vi "Rotation_CreateAngleDegrees.vi"(11 "Angle_Degrees":dbl) -> (3 "ROTATION":T1 {"SIN" format="%13.4f"; "COS" format="%13.4f"; "VALUE" format="%13.4f"})   [LabVIEW 2019, in "Trajectory_Library.lvlib"]
doc: "Constructs a Rotation2d with the given angle value in degrees. \nParmeters:\n - value - The value of the angle in degrees..\n\nReturns\n - rotation data structure"
uses:
  Trajectory_Library.lvlib
  ROTATION2D.ctl
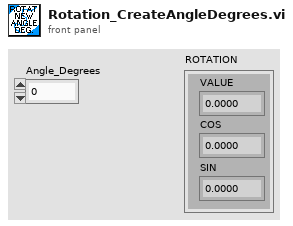
[diagram p1: front panel]
types:
  T1 = typedef "Trajectory_Library.lvlib/ROTATION2D.ctl" = cluster{"VALUE":dbl, "COS":dbl, "SIN":dbl}
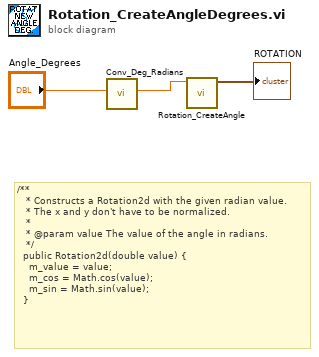
[diagram p0: block diagram]
diagram:
  # "/**\n   * Constructs a Rotation2d with the given radian value.\n   * The x and y don't have to be normalized.\n   *\n   * @param value The value of the angle in radians.\n   */\n  public Rotation2d(double value) {\n    m_value = value;\n    m_cos = Math.cos(value);\n    m_sin = Math.sin(value);\n  }"
  n1 = call "Conv_Deg_Radians.vi"("Degress"="Angle_Degrees") -> ("Radians"=w2:dbl)  [unwired: 10 in]
  n2 = call "Rotation_CreateAngle.vi"("Angle"=w2) -> ("ROTATION"=→"ROTATION":T1)  [unwired: 10 in]
